vi "font.vi"(8 "Error In":errorcluster, 10 "className (\"QWidget\")":string="QWidget", 11 "LQWidgetEngine In":refnum<class "LQWidgetEngine.lvclass">) -> (0 "Error Out":errorcluster, 2 "Value":refnum<class "QFont.lvclass">, 3 "LQWidgetEngine Out":refnum<class "LQWidgetEngine.lvclass">)   [LabVIEW 2014, in "LQWidgetEngine.lvclass"]
doc: "LabVIEW-specific documentation is not yet available. See <b>https://doc.qt.io/qt-5/qapplication.html#font</b>"
uses:
  LQWidgetEngine.lvclass
  Qt GUI/QFont/QFont.lvclass
  LQ Core/LQIdentity/LQIdentity.lvclass/LQIdentity.ctl
  LQ Core/LQSerialData/LQSerialData.lvclass/LQSerialData.ctl
  LQ Core/LQ Core.lvlib
  LQ Core/LQIdentity/LQIdentity.lvclass
  LQ Core/LQSerialData/LQSerialData.lvclass
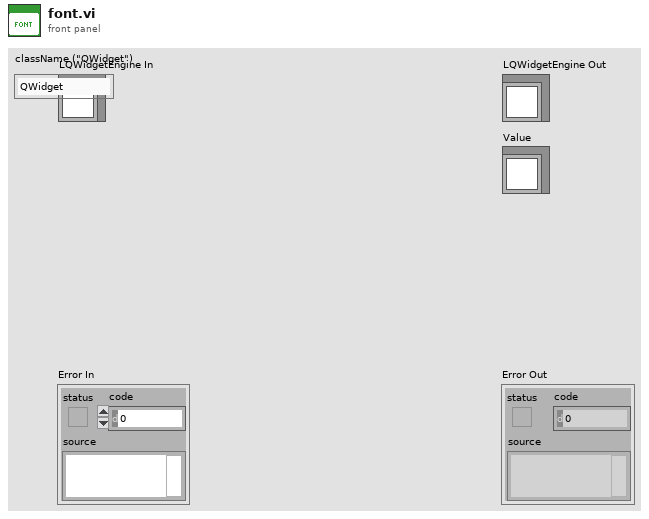
[diagram p1: front panel]
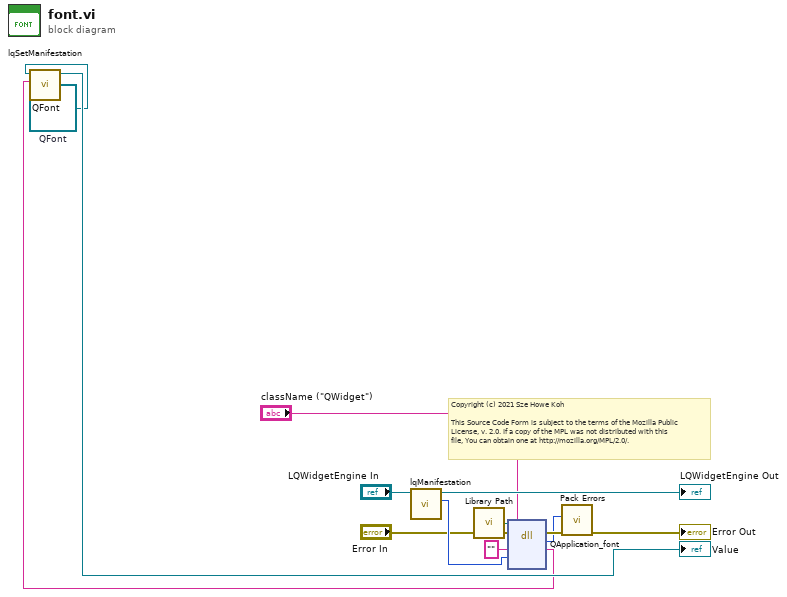
[diagram p0: block diagram]
diagram:
  w2 = refnum<class "QFont.lvclass"> refnum  # QFont
  # "Copyright (c) 2021 Sze Howe Koh\n\nThis Source Code Form is subject to the terms of the Mozilla Public\nLicense, v. 2.0. If a copy of the MPL was not distributed with this\nfile, You can obtain one at http://mozilla.org/MPL/2.0/."
  n1 = call "lqManifestation.vi"("LQIdentity in"="LQWidgetEngine In") -> ("Manifestation"=w9:u64, "LQIdentity out"=→"LQWidgetEngine Out":refnum<class "LQWidgetEngine.lvclass">)  [unwired: 9 in]
  n2 = call "Library Path.vi"() -> ("Library Path"=w10:path)
  n3 = dll-call lib="?" fn="QApplication_font"(path in=w10, error in="Error In", "_retVal"="" ("retVal"), "_instance"=w9, "className"="className (\"QWidget\")") -> (error out=w7:errorcluster, w5:i32, "_retVal"=w3:string)  [unwired: 3 in, 1 out]
  n4 = call "lqSetManifestation.vi"("Manifestation"=w3, "LQSerialData in"=w2) -> ("LQSerialData out"=→"Value":refnum<class "QFont.lvclass">)  [unwired: 8 in, 1 out]
  n5 = call "Pack Errors.vi"("Error In"=w7, "Error Code"=w5) -> ("Error Out"=→"Error Out":errorcluster)  [unwired: 9 in]
